vi "PCAOM_control_v6.vi"() -> ()   [LabVIEW 2012]
uses:
  <vilib>/DAQmx/write.llb/DAQmx Write (Digital Bool 1Line 1Point).vi
  <vilib>/DAQmx/create/channels.llb/DAQmx Create Channel (DO-Digital Output).vi
  <vilib>/DAQmx/miscellaneous.llb/DAQmx Fill In Error Info.vi
panel:
  out "error out 2":errorcluster
  in  "Array":dbl[](array[numeric])
  in  "time between (ms)":u32
  in  "stimulation time  (ms)":u32=500
  in  "Optopatch":bool
  out "DAQ err 3":errorcluster
  in  "488 shutter":bool
  in  "488 shutter line":tag="Dev1/port0/line15"
  out "DAQ err 2":errorcluster
  in  "532 shutter":bool
  in  "532 shutter line":tag="Dev1/port0/line14"
  out "DAQ err":errorcluster
  in  "637 shutter":bool
  in  "637 shutter line":tag="Dev1/port0/line8"
  in  "stop":bool
  in  "blue":bool
  in  "green":bool
  in  "yellow":bool
  in  "orange":bool
  in  "red":bool
  out "concatenated string":string="ch3\r\nfr 80.25\r\nam 680\r\noff\r\n"
  in  "COM port":refnum<visa-resource-name>="COM3"
  in  "Amplitude":string[](array[string])=["am 610", "am 455", "am 386", "am 485", "am 670"]
  in  "Frequency":string[](array[string])=["fr 54.015", "fr 57.795", "fr 62.051", "fr 68.05", "fr 80.27"]
  in  "Channel":string[](array[string])=["ch2", "ch3", "ch5", "ch4", "ch1"]
  out "error out":errorcluster
  # "Max_Amp_OlympusII"
  # "am 500"
  # "637 nm"
  # "594 nm"
  # "561 nm"
  # "532 nm"
  # "am 470"
  # "488 nm"
  # "am 680"
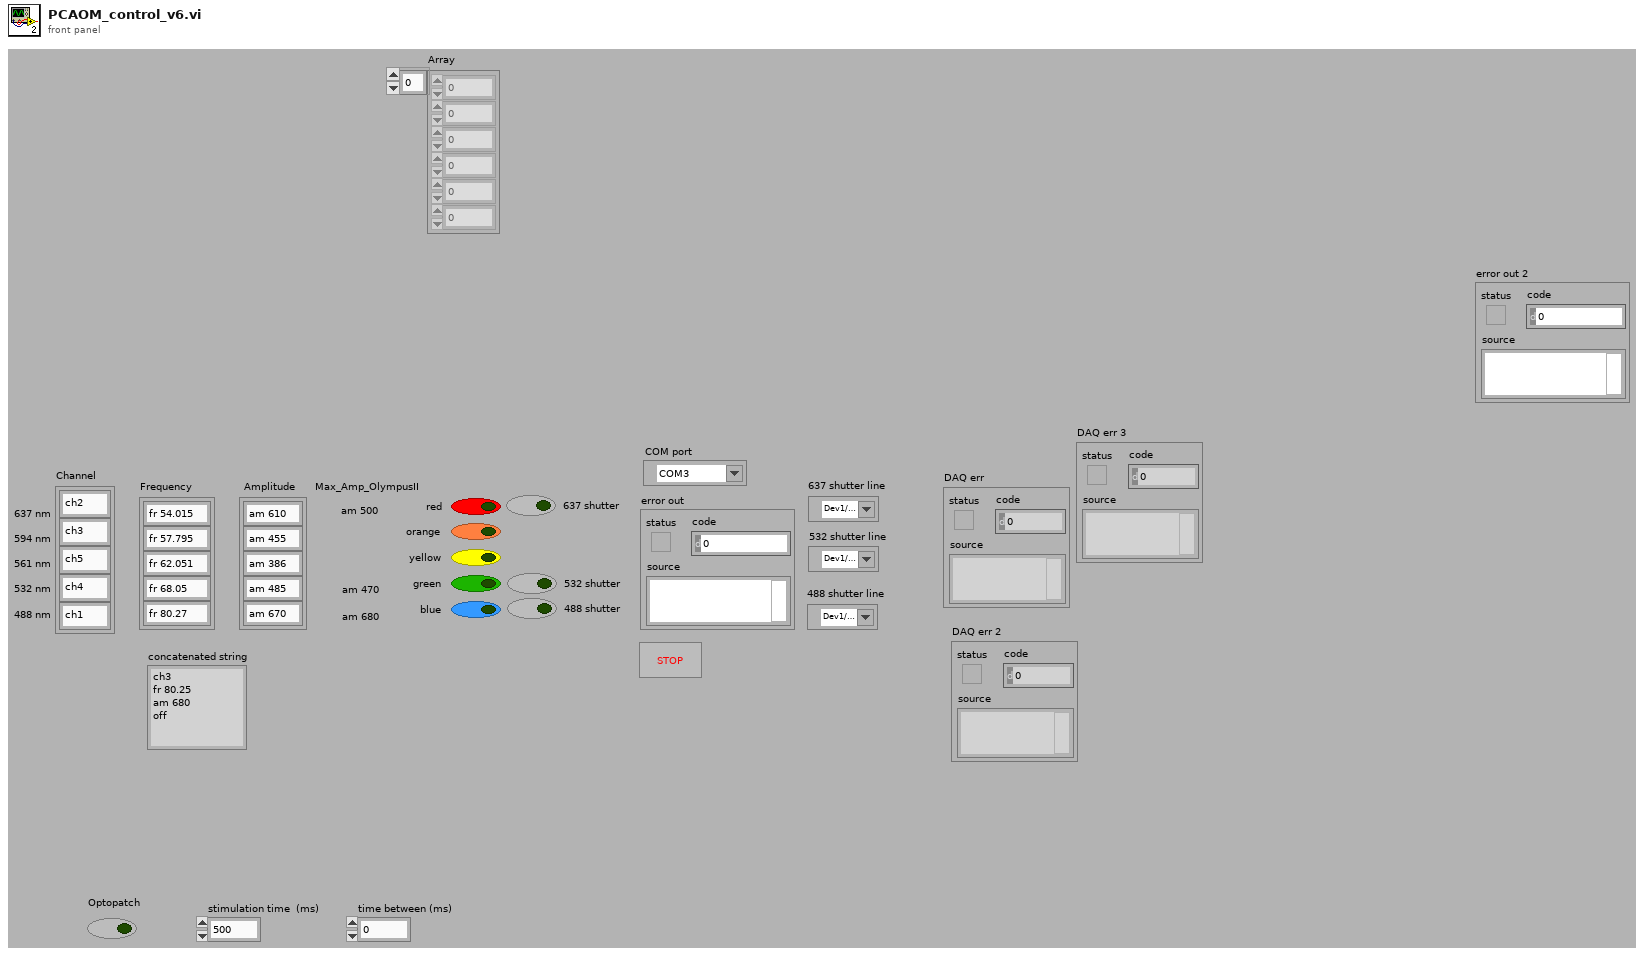
[diagram p1: front panel]
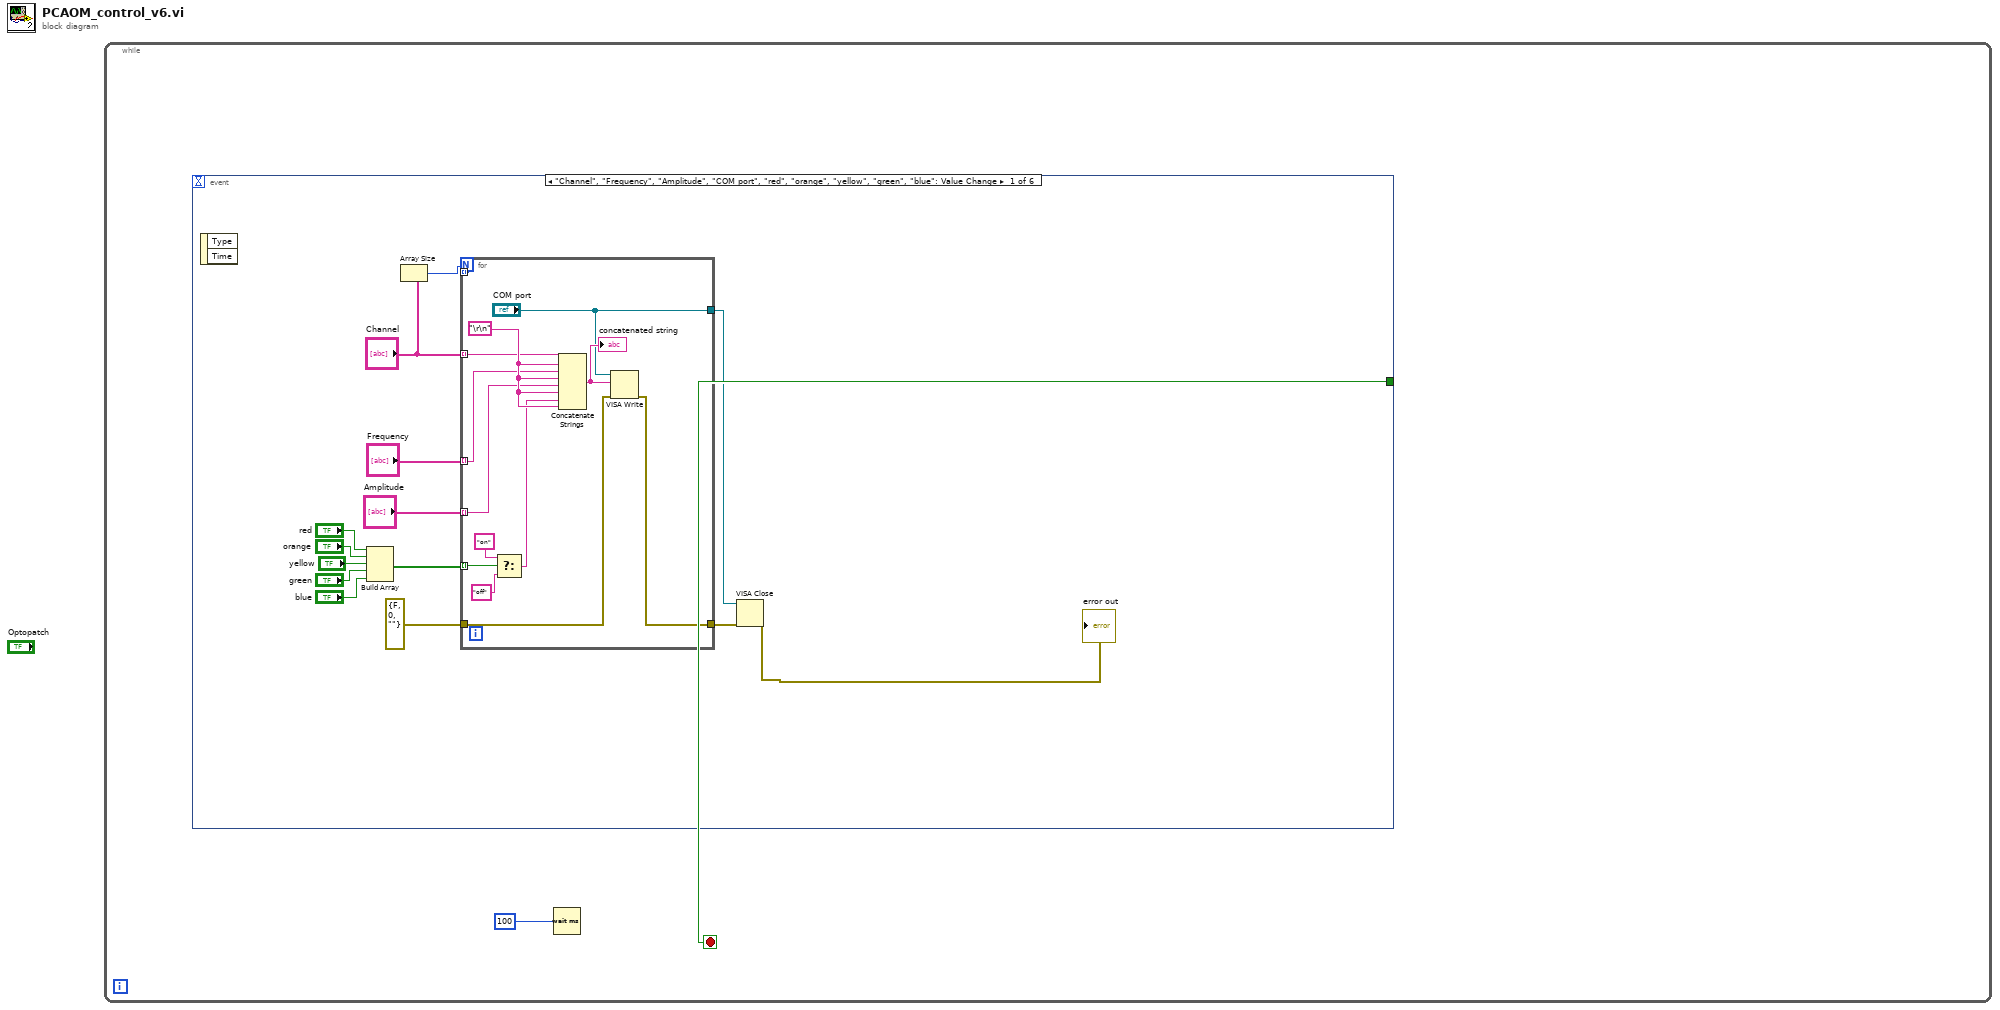
[diagram p0: block diagram]
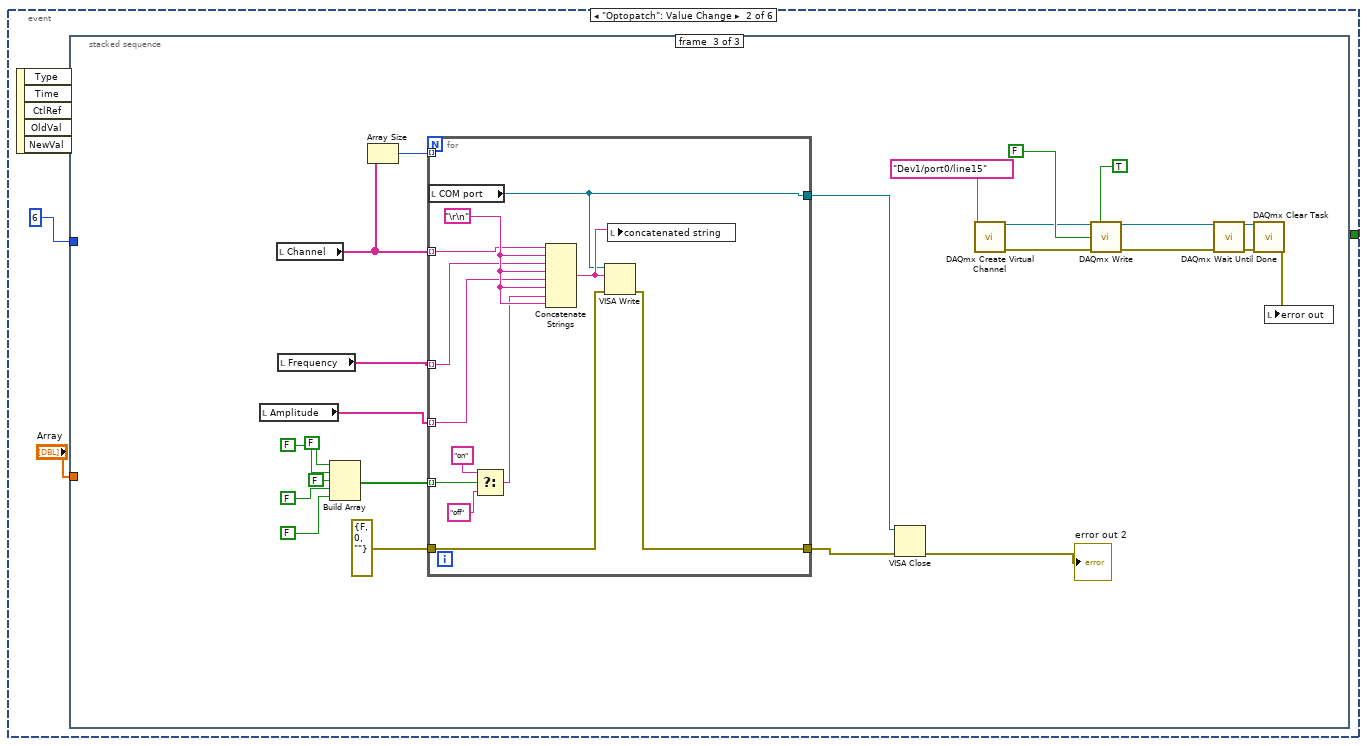
[diagram p2: hidden frame]
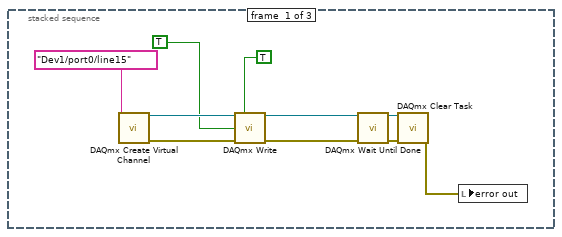
[diagram p3: hidden frame]
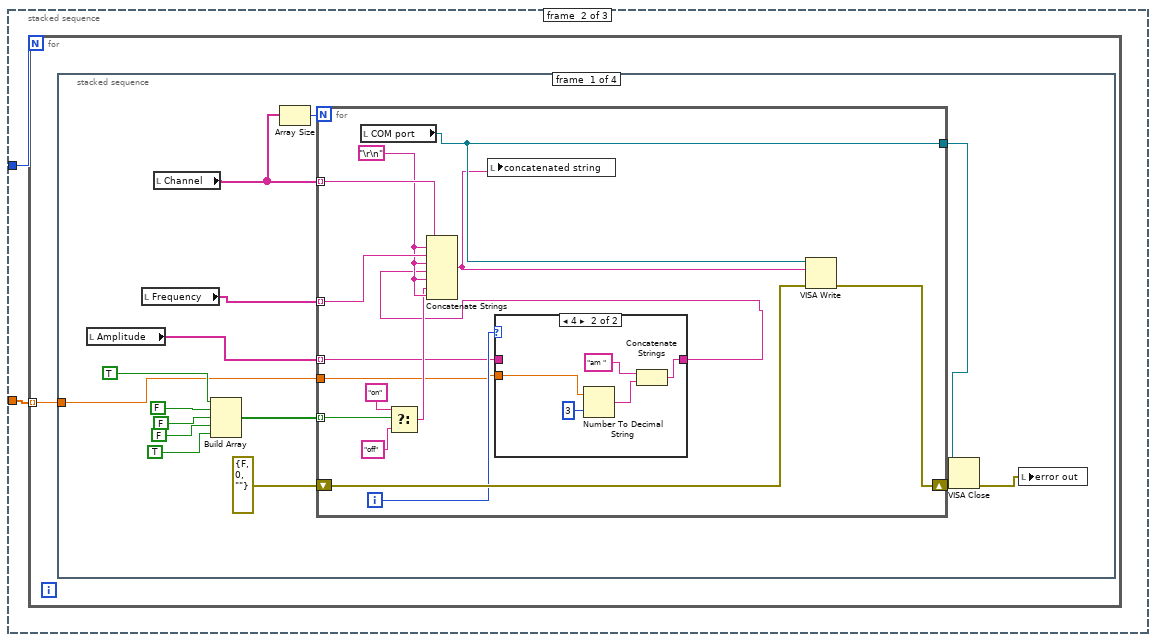
[diagram p4: hidden frame]
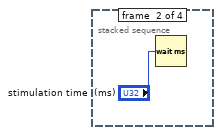
[diagram p6: hidden frame]
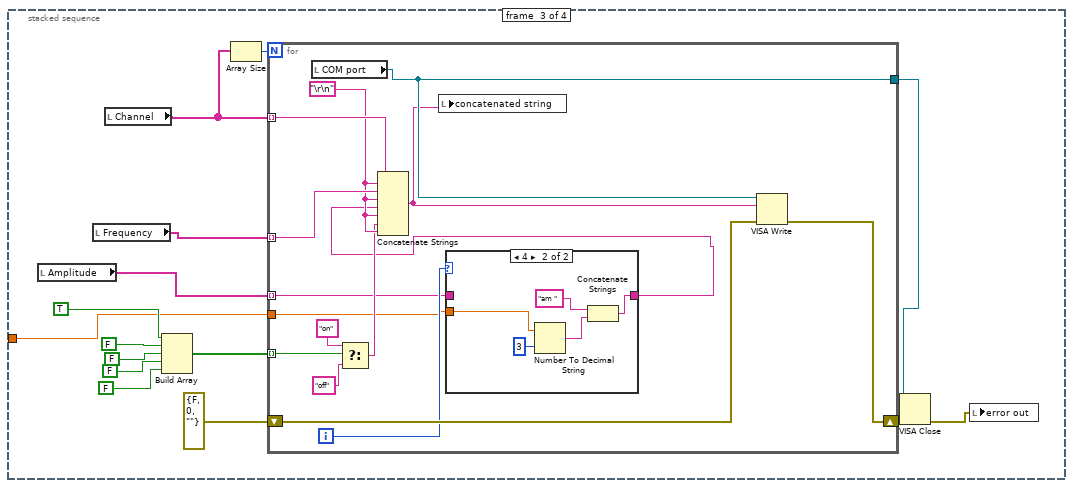
[diagram p7: hidden frame]
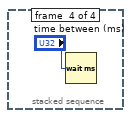
[diagram p9: hidden frame]
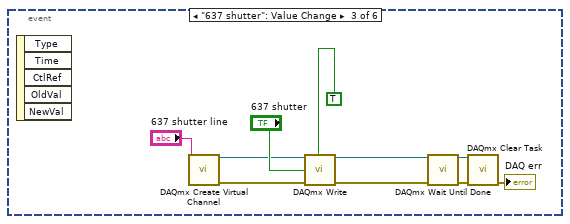
[diagram p10: hidden frame]
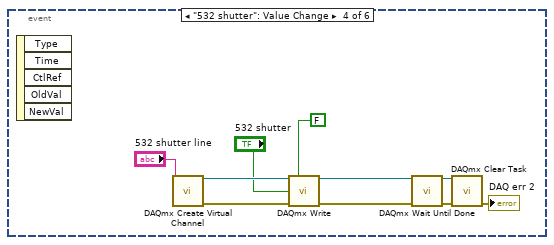
[diagram p11: hidden frame]
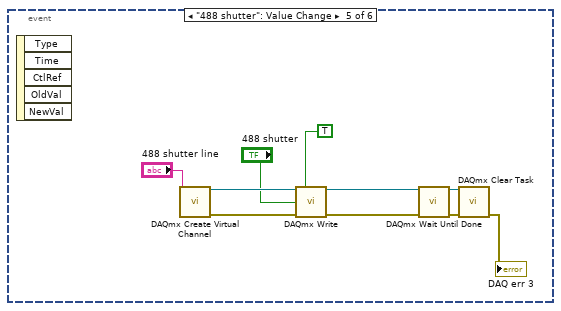
[diagram p12: hidden frame]
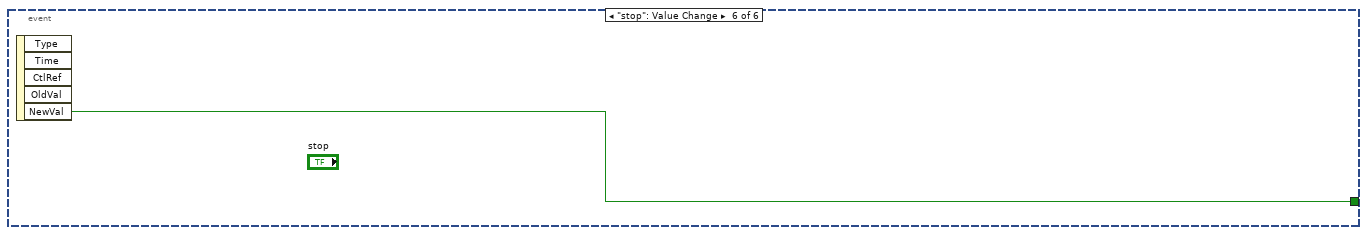
[diagram p13: hidden frame]
diagram:
  n1 = while {
    stop <- w1 stop-if-true
    n2 = event shown="[0] \"Channel\", \"Frequency\", \"Amplitude\", \"COM port\", \"red\", \"orange\", \"yellow\", \"green\", \"blue\": Value Change" {
      selector: _ -> [_ _ _ _ _ _]
      dyn-events: _ -> [_ _ _ _ _ _]
      timeout: _ -> [_ _ _ _ _ _]
      tunnel: [_ _ _ _ _ w186] -> w1
      event "Channel", "Frequency", "Amplitude", "COM port", "red", "orange", "yellow", "green", "blue": Value Change {
        n3 = event-data() -> ()  [unwired: 1 in, 2 out]
        n4 = Build Array("red", "orange", "yellow", "green", "blue") -> (w4:bool[])
        n5 = Array Size(array="Channel") -> (size(s)=w3:i32)
        n6 = for {
          N: w3 -> [w17]
          tunnel: "Channel" -> [w24] mode=indexing
          tunnel: "Frequency" -> [w23] mode=indexing
          tunnel: "Amplitude" -> [w22] mode=indexing
          tunnel: errorcluster {"status"=FALSE, "code"=0, "source"=""} ("error in (no error)") -> [w21]
          tunnel: [w20] -> w6
          tunnel: ["COM port"] -> w5
          tunnel: w4 -> [w18] mode=indexing
          tunnel: [w17] -> _ mode=indexing
          w29 = "\r\n"
          n7 = Select(t="on", s=w18, f="off") -> (s? t:f=w27:string)
          n8 = Concatenate Strings(w24, w29, w23, w29, w22, w29, w27, w29) -> (w28:string)
          "concatenated string" <- w28
          n9 = VISA Write(VISA resource name="COM port", write buffer=w28, error in (no error)=w21) -> (error out=w20:errorcluster)  [unwired: 2 out]
        }
        n10 = VISA Close(VISA resource name=w5, error in (no error)=w6) -> (error out=→"error out":errorcluster)
      }
      event "Optopatch": Value Change {
        n11 = event-data() -> ()  [unwired: 1 in, 5 out]
        n12 = stacked-sequence {
          tunnel: 6 -> [_ w43 _]
          tunnel: "Array" -> [_ w42 _]
          frame #0 {
            n13 = call-poly <vilib>:"DAQmx Create Virtual Channel.vi"("lines"=tag "Dev1/port0/line15" ("488 shutter line 2")) -> ("task out"=w40:refnum<k21>, "error out"=w37:errorcluster)  [unwired: 13 in]
            n14 = call-poly <vilib>:"DAQmx Write.vi"("task/channels in"=w40, "auto start"=TRUE, "data"=TRUE ("488 shutter 2"), "error in"=w37) -> ("task out"=w36:refnum<k21>, "error out"=w35:errorcluster)  [unwired: 9 in, 1 out]
            n15 = call <vilib>:"DAQmx Wait Until Done.vi"("task/channels in"=w36, "error in"=w35) -> ("task out"=w34:refnum<k21>, "error out"=w33:errorcluster)  [unwired: 12 in]
            n16 = call <vilib>:"DAQmx Clear Task.vi"("task in"=w34, "error in"=w33) -> ("error out"=w32:errorcluster)  [unwired: 13 in]
            n17 = local write "error out"(w32) -> ()
          }
          frame #1 {
            n18 = for {
              N: w43 -> [_]
              tunnel: w42 -> [w44] mode=indexing
              n19 = stacked-sequence {
                tunnel: w44 -> [w45 _ w82 _]
                frame #0 {
                  n20 = local read "Amplitude"() -> (w48:string[])
                  n21 = local read "Frequency"() -> (w49:string[])
                  n22 = local read "Channel"() -> (w50:string[])
                  n23 = Build Array(TRUE, FALSE ("orange 2"), FALSE ("yellow 2"), FALSE ("green 2"), TRUE ("blue 2")) -> (w52:bool[])
                  n24 = Array Size(array=w50) -> (size(s)=w51:i32)
                  n25 = for {
                    N: w51 -> [_]
                    tunnel: w50 -> [w74] mode=indexing
                    tunnel: w49 -> [w73] mode=indexing
                    tunnel: w48 -> [w61] mode=indexing
                    shift-right: [w70] -> w58
                    shift-left: errorcluster {"status"=FALSE, "code"=0, "source"=""} ("error in (no error)") -> [w71]
                    tunnel: [w65] -> w57
                    tunnel: w52 -> [w69] mode=indexing
                    tunnel: w45 -> [w62]
                    i -> [w63]
                    w72 = "\r\n"
                    n26 = local read "COM port"() -> (w65:refnum<visa-resource-name>)
                    n27 = Select(t="on", s=w69, f="off") -> (s? t:f=w68:string)
                    n28 = case shown="4" w63 {
                      tunnel: w62 -> [_ w80]
                      tunnel: w61 -> [w75 _]
                      tunnel: [w75 w78] -> w60
                      frame 0, Default {
                      }
                      frame 4 {
                        n29 = Number To Decimal String(number=w80, width (-)=i16 3) -> (decimal integer string=w76:string)
                        n30 = Concatenate Strings("am ", w76) -> (w78:string)
                      }
                    }
                    n31 = Concatenate Strings(w74, w72, w73, w72, w60, w72, w68, w72) -> (w64:string)
                    n32 = local write "concatenated string"(w64) -> ()
                    n33 = VISA Write(VISA resource name=w65, write buffer=w64, error in (no error)=w71) -> (error out=w70:errorcluster)  [unwired: 2 out]
                  }
                  n34 = VISA Close(VISA resource name=w57, error in (no error)=w58) -> (error out=w47:errorcluster)
                  n35 = local write "error out"(w47) -> ()
                }
                frame #1 {
                  n36 = Wait (ms)(milliseconds to wait="stimulation time  (ms)") -> ()  [unwired: 1 out]
                }
                frame #2 {
                  n37 = local read "Amplitude"() -> (w85:string[])
                  n38 = local read "Frequency"() -> (w86:string[])
                  n39 = local read "Channel"() -> (w87:string[])
                  n40 = Build Array(TRUE, FALSE ("orange 2"), FALSE ("yellow 2"), FALSE ("green 2"), FALSE ("blue 2")) -> (w89:bool[])
                  n41 = Array Size(array=w87) -> (size(s)=w88:i32)
                  n42 = for {
                    N: w88 -> [_]
                    tunnel: w87 -> [w111] mode=indexing
                    tunnel: w86 -> [w110] mode=indexing
                    tunnel: w85 -> [w98] mode=indexing
                    shift-right: [w107] -> w95
                    shift-left: errorcluster {"status"=FALSE, "code"=0, "source"=""} ("error in (no error)") -> [w108]
                    tunnel: [w102] -> w94
                    tunnel: w89 -> [w106] mode=indexing
                    tunnel: w82 -> [w99]
                    i -> [w100]
                    w109 = "\r\n"
                    n43 = local read "COM port"() -> (w102:refnum<visa-resource-name>)
                    n44 = Select(t="on", s=w106, f="off") -> (s? t:f=w105:string)
                    n45 = case shown="4" w100 {
                      tunnel: w99 -> [_ w117]
                      tunnel: w98 -> [w112 _]
                      tunnel: [w112 w115] -> w97
                      frame 0, Default {
                      }
                      frame 4 {
                        n46 = Number To Decimal String(number=w117, width (-)=i16 3) -> (decimal integer string=w113:string)
                        n47 = Concatenate Strings("am ", w113) -> (w115:string)
                      }
                    }
                    n48 = Concatenate Strings(w111, w109, w110, w109, w97, w109, w105, w109) -> (w101:string)
                    n49 = local write "concatenated string"(w101) -> ()
                    n50 = VISA Write(VISA resource name=w102, write buffer=w101, error in (no error)=w108) -> (error out=w107:errorcluster)  [unwired: 2 out]
                  }
                  n51 = VISA Close(VISA resource name=w94, error in (no error)=w95) -> (error out=w84:errorcluster)
                  n52 = local write "error out"(w84) -> ()
                }
                frame #3 {
                  n53 = Wait (ms)(milliseconds to wait="time between (ms)") -> ()  [unwired: 1 out]
                }
              }
            }
          }
          frame #2 {
            n54 = local read "Amplitude"() -> (w132:string[])
            n55 = local read "Channel"() -> (w129:string[])
            n56 = local read "Frequency"() -> (w131:string[])
            n57 = Build Array(FALSE ("red 2"), FALSE ("orange 2"), FALSE ("yellow 2"), FALSE ("green 2"), FALSE ("blue 2")) -> (w135:bool[])
            n58 = Array Size(array=w129) -> (size(s)=w130:i32)
            n59 = for {
              N: w130 -> [w146]
              tunnel: w131 -> [w151] mode=indexing
              tunnel: w132 -> [w150] mode=indexing
              tunnel: errorcluster {"status"=FALSE, "code"=0, "source"=""} ("error in (no error)") -> [w149]
              tunnel: [w148] -> w136
              tunnel: [w143] -> w134
              tunnel: w135 -> [w147] mode=indexing
              tunnel: [w146] -> _ mode=indexing
              tunnel: w129 -> [w144] mode=indexing
              w155 = "\r\n"
              n60 = local read "COM port"() -> (w143:refnum<visa-resource-name>)
              n61 = Select(t="on", s=w147, f="off") -> (s? t:f=w154:string)
              n62 = Concatenate Strings(w144, w155, w151, w155, w150, w155, w154, w155) -> (w145:string)
              n63 = VISA Write(VISA resource name=w143, write buffer=w145, error in (no error)=w149) -> (error out=w148:errorcluster)  [unwired: 2 out]
              n64 = local write "concatenated string"(w145) -> ()
            }
            n65 = VISA Close(VISA resource name=w134, error in (no error)=w136) -> (error out=→"error out 2":errorcluster)
            n66 = call-poly <vilib>:"DAQmx Create Virtual Channel.vi"("lines"=tag "Dev1/port0/line15" ("488 shutter line 2")) -> ("task out"=w121:refnum<k21>, "error out"=w124:errorcluster)  [unwired: 13 in]
            n67 = call-poly <vilib>:"DAQmx Write.vi"("task/channels in"=w121, "auto start"=TRUE, "data"=FALSE ("488 shutter 2"), "error in"=w124) -> ("task out"=w125:refnum<k21>, "error out"=w126:errorcluster)  [unwired: 9 in, 1 out]
            n68 = call <vilib>:"DAQmx Wait Until Done.vi"("task/channels in"=w125, "error in"=w126) -> ("task out"=w127:refnum<k21>, "error out"=w128:errorcluster)  [unwired: 12 in]
            n69 = call <vilib>:"DAQmx Clear Task.vi"("task in"=w127, "error in"=w128) -> ("error out"=w119:errorcluster)  [unwired: 13 in]
            n70 = local write "error out"(w119) -> ()
          }
        }
      }
      event "637 shutter": Value Change {
        n71 = event-data() -> ()  [unwired: 1 in, 5 out]
        n72 = call-poly <vilib>:"DAQmx Create Virtual Channel.vi"("lines"="637 shutter line") -> ("task out"=w157:refnum<k21>, "error out"=w160:errorcluster)  [unwired: 13 in]
        n73 = call-poly <vilib>:"DAQmx Write.vi"("task/channels in"=w157, "auto start"=TRUE, "data"="637 shutter", "error in"=w160) -> ("task out"=w161:refnum<k21>, "error out"=w162:errorcluster)  [unwired: 9 in, 1 out]
        n74 = call <vilib>:"DAQmx Wait Until Done.vi"("task/channels in"=w161, "error in"=w162) -> ("task out"=w163:refnum<k21>, "error out"=w164:errorcluster)  [unwired: 12 in]
        n75 = call <vilib>:"DAQmx Clear Task.vi"("task in"=w163, "error in"=w164) -> ("error out"=→"DAQ err":errorcluster)  [unwired: 13 in]
      }
      event "532 shutter": Value Change {
        n76 = event-data() -> ()  [unwired: 1 in, 5 out]
        n77 = call-poly <vilib>:"DAQmx Create Virtual Channel.vi"("lines"="532 shutter line") -> ("task out"=w174:refnum<k21>, "error out"=w171:errorcluster)  [unwired: 13 in]
        n78 = call-poly <vilib>:"DAQmx Write.vi"("task/channels in"=w174, "auto start"=FALSE, "data"="532 shutter", "error in"=w171) -> ("task out"=w170:refnum<k21>, "error out"=w169:errorcluster)  [unwired: 9 in, 1 out]
        n79 = call <vilib>:"DAQmx Wait Until Done.vi"("task/channels in"=w170, "error in"=w169) -> ("task out"=w168:refnum<k21>, "error out"=w167:errorcluster)  [unwired: 12 in]
        n80 = call <vilib>:"DAQmx Clear Task.vi"("task in"=w168, "error in"=w167) -> ("error out"=→"DAQ err 2":errorcluster)  [unwired: 13 in]
      }
      event "488 shutter": Value Change {
        n81 = event-data() -> ()  [unwired: 1 in, 5 out]
        n82 = call-poly <vilib>:"DAQmx Create Virtual Channel.vi"("lines"="488 shutter line") -> ("task out"=w184:refnum<k21>, "error out"=w181:errorcluster)  [unwired: 13 in]
        n83 = call-poly <vilib>:"DAQmx Write.vi"("task/channels in"=w184, "auto start"=TRUE, "data"="488 shutter", "error in"=w181) -> ("task out"=w180:refnum<k21>, "error out"=w179:errorcluster)  [unwired: 9 in, 1 out]
        n84 = call <vilib>:"DAQmx Wait Until Done.vi"("task/channels in"=w180, "error in"=w179) -> ("task out"=w178:refnum<k21>, "error out"=w177:errorcluster)  [unwired: 12 in]
        n85 = call <vilib>:"DAQmx Clear Task.vi"("task in"=w178, "error in"=w177) -> ("error out"=→"DAQ err 3":errorcluster)  [unwired: 13 in]
      }
      event "stop": Value Change {
        n86 = event-data() -> ("NewVal"=w186:bool)  [unwired: 1 in, 4 out]
      }
    }
    n87 = Wait (ms)(milliseconds to wait=u32 100) -> ()  [unwired: 1 out]
  }
